vi "Read Roles.vi"(8 "error in (no error)":errorcluster, 11 "PreparePenaltyAllyPlayVSS in":refnum<class "PreparePenaltyAllyPlayVSS.lvclass">) -> (0 "error out":errorcluster, 2 "Roles":T1, 3 "PreparePenaltyAllyPlayVSS out":refnum<class "PreparePenaltyAllyPlayVSS.lvclass">)   [LabVIEW 2023, in "PreparePenaltyAllyPlayVSS.lvclass"]
uses:
  PreparePenaltyAllyPlayVSS.lvclass
  HaltRole_class/HaltRole.lvclass
  AttackerAimGoalRoleVSS_class/AttackerAimGoalRoleVSS.lvclass
  PreparePenaltyAllyPlayVSS.lvclass/PreparePenaltyAllyPlayVSS.ctl
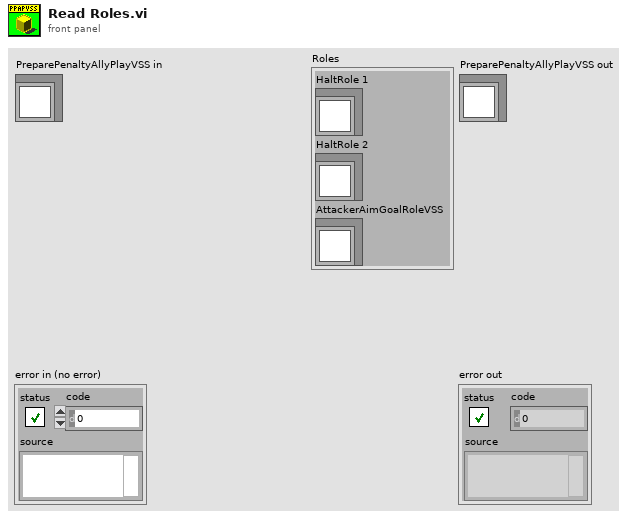
[diagram p1: front panel]
types:
  T1 = cluster{"HaltRole 1":refnum<class "HaltRole.lvclass">, "HaltRole 2":refnum<class "HaltRole.lvclass">, "AttackerAimGoalRoleVSS":refnum<class "AttackerAimGoalRoleVSS.lvclass">}
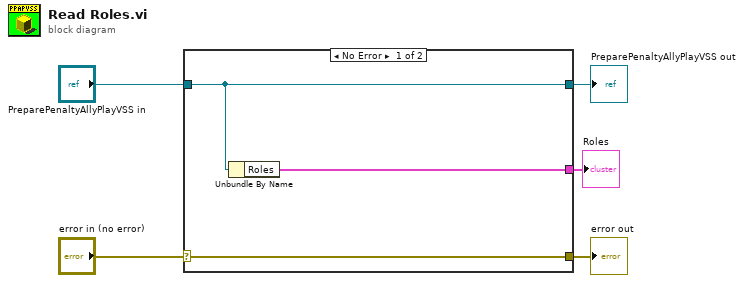
[diagram p0: block diagram]
diagram:
  n1 = case shown="No Error" "error in (no error)" {
    selector: "error in (no error)" -> [w8 w9]
    tunnel: [w8 w9] -> w4
    tunnel: [w7 w10] -> w2
    tunnel: "PreparePenaltyAllyPlayVSS in" -> [w7 w10]
    tunnel: [w6 _] -> w1
    frame No Error {
      n2 = Unbundle By Name(w7) -> ("Roles"=w6:T1)
    }
    frame Error {
    }
  }
  "error out" <- w4
  "PreparePenaltyAllyPlayVSS out" <- w2
  "Roles" <- w1
